vi "Image_Actions_V3.vi"(0 "Image Size (Pixels)":T2={"Pixels Per Line"=128, "Number of Lines"=128}, 2 "Mode":u16(ring) items=["Write", "Read"], 7 "Number of Channels":i32, 11 "Action":string) -> (4 "Image REFs OUT":T1[](array[typedef]), 15 "Image Names OUT":string[](array[string]))   [LabVIEW 2014]
uses:
  <vilib>/vision/Image Controls.llb/IMAQ Image.ctl
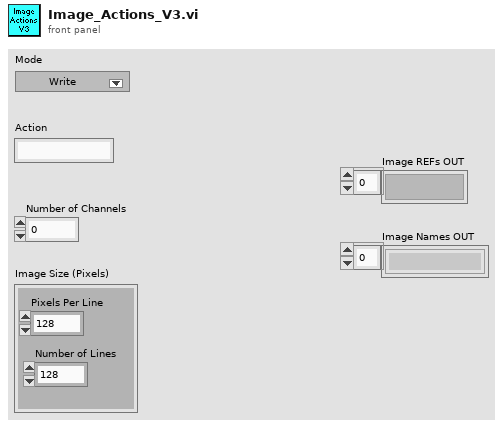
[diagram p1: front panel]
types:
  T1 = typedef "IMAQ Image.ctl" = refnum<image>
  T2 = cluster{"Pixels Per Line":i32, "Number of Lines":i32}
  T3 = typedef "Image Type" = u32
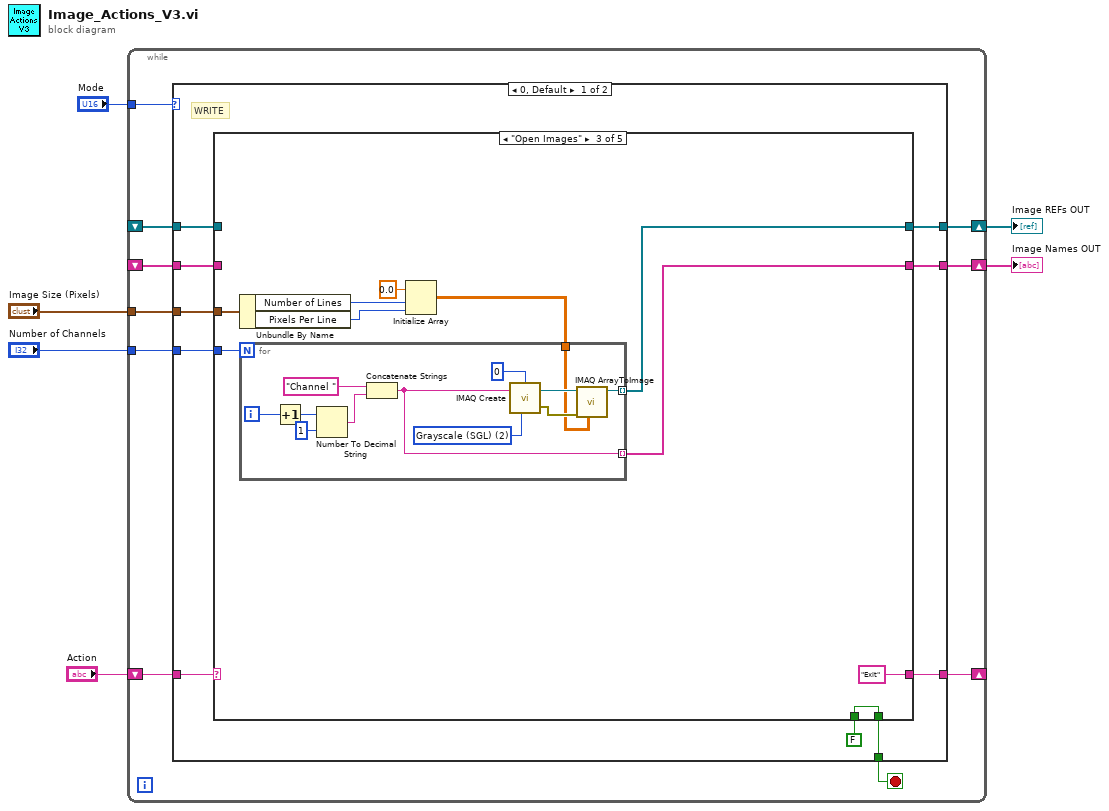
[diagram p0: block diagram]
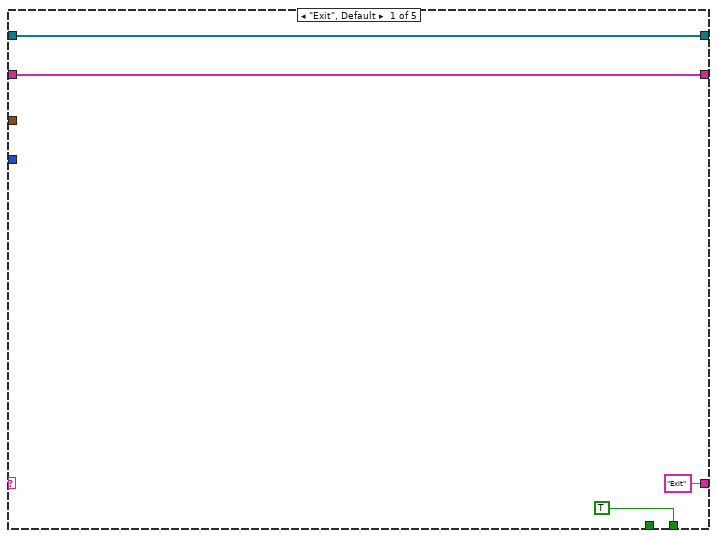
[diagram p2: hidden frame]
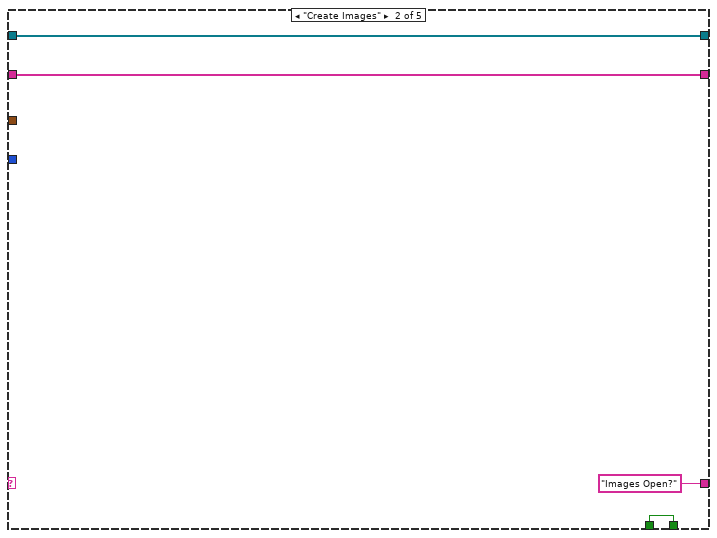
[diagram p3: hidden frame]
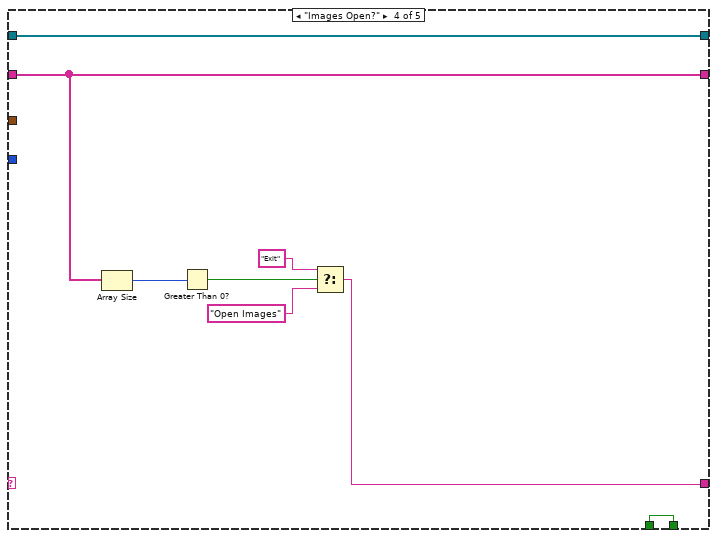
[diagram p4: hidden frame]
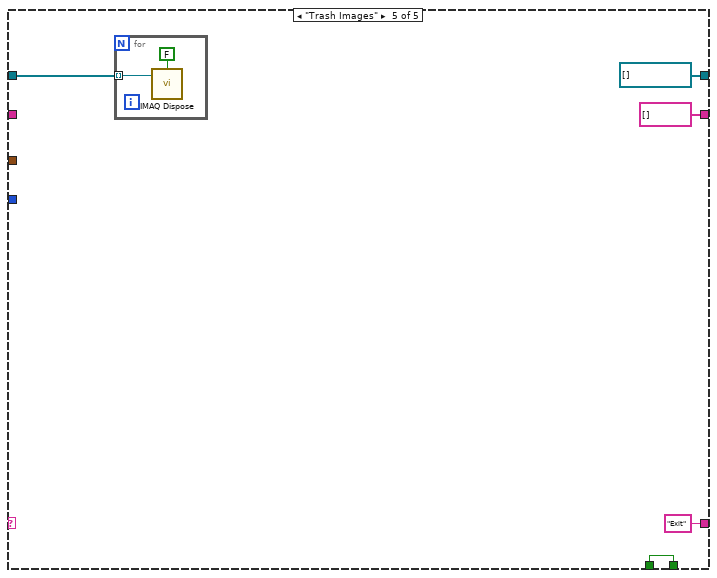
[diagram p5: hidden frame]
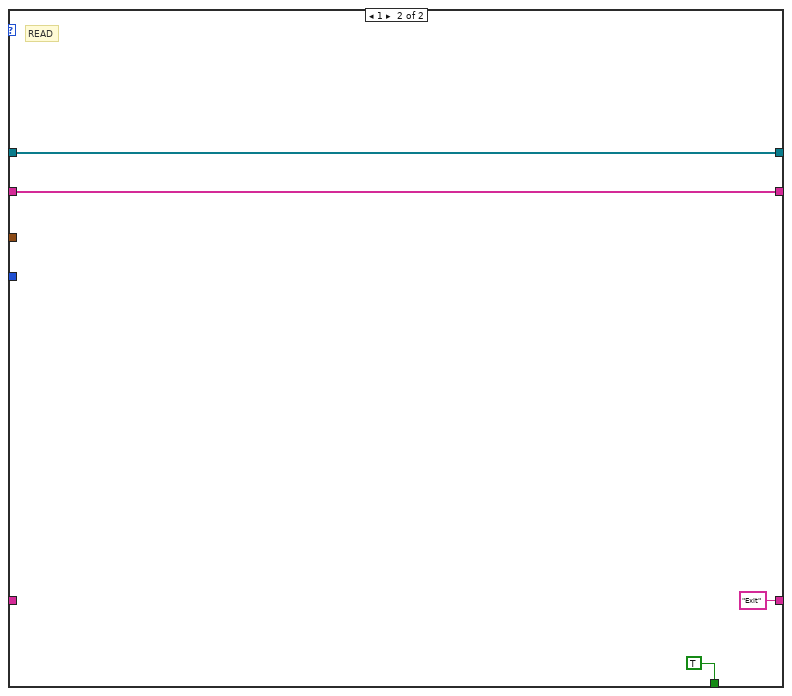
[diagram p6: hidden frame]
diagram:
  n1 = while {
    tunnel: "Mode" -> [w16]
    shift-right: [w7] -> _
    shift-left: "Action" -> [w14]
    shift-right: [w11] -> w2
    shift-left: _ -> [w9]
    tunnel: "Number of Channels" -> [w13]
    tunnel: "Image Size (Pixels)" -> [w12]
    shift-right: [w10] -> w1
    shift-left: _ -> [w8]
    stop <- w15 stop-if-true
    n2 = case shown="0, Default" w16 {
      tunnel: [w21 TRUE] -> w15
      tunnel: w14 -> [w26 _]
      tunnel: w13 -> [w25 _]
      tunnel: w12 -> [w24 _]
      tunnel: [w23 w74] -> w11
      tunnel: [w22 w73] -> w10
      tunnel: w9 -> [w18 w74]
      tunnel: w8 -> [w17 w73]
      tunnel: [w19 "Exit"] -> w7
      frame 0, Default {
        # "WRITE"
        n3 = case shown="\"Open Images\"" w26 {
          tunnel: w25 -> [_ _ w44 _ _]
          tunnel: w24 -> [_ _ w43 _ _]
          tunnel: [w28 w32 w38 w63 T1[] []] -> w23
          tunnel: [w27 w31 w37 w62 string[] []] -> w22
          tunnel: [TRUE w34 w36 w64 w67] -> w21
          tunnel: FALSE -> [_ w34 w36 w64 w67]
          tunnel: ["Exit" "Images Open?" "Exit" w59 "Exit"] -> w19
          tunnel: w18 -> [w28 w32 _ w63 w65]
          tunnel: w17 -> [w27 w31 _ w62 _]
          frame "Exit", Default {
          }
          frame "Create Images" {
          }
          frame "Open Images" {
            n4 = Unbundle By Name(w43) -> ("Number of Lines"=w41:i32, "Pixels Per Line"=w42:i32)
            n5 = Initialize Array(sgl 0.0 ("element"), w41, w42) -> (w39:sgl[][])
            n6 = for {
              N: w44 -> [_]
              tunnel: w39 -> [w48]
              tunnel: [w46] -> w38 mode=indexing
              tunnel: [w45] -> w37 mode=indexing
              i -> [w47]
              w52 = T3 2 items=["Grayscale (U8)", "Grayscale (I16)", "Grayscale (SGL)", "Complex (CSG)", "RGB (U32)", "HSL (U32)", "RGB (U64)", "Grayscale (U16)"] ("Image Type")
              n7 = Increment(x=w47) -> (x+1=w54:i32)
              n8 = Number To Decimal String(number=w54, width (-)=i16 1) -> (decimal integer string=w51:string)
              n9 = Concatenate Strings("Channel ", w51) -> (w45:string)
              n10 = call "IMAQ Create"("Border Size"=0, "Image Name"=w45, "Image Type"=w52) -> ("New Image"=w53:T1, "error out"=w56:errorcluster)  [unwired: 2 in]
              n11 = call "IMAQ ArrayToImage"("Image Pixels (Float)"=w48, "error in (no error)"=w56, "Image"=w53) -> ("Image Out"=w46:T1)  [unwired: 7 in, 1 out]
            }
          }
          frame "Images Open?" {
            n12 = Array Size(array=w62) -> (size(s)=w61:i32)
            n13 = Greater Than 0?(x=w61) -> (x > 0?=w60:bool)
            n14 = Select(t="Exit", s=w60, f="Open Images") -> (s? t:f=w59:string)
          }
          frame "Trash Images" {
            n15 = for {
              tunnel: w65 -> [w71] mode=indexing
              n16 = call "IMAQ Dispose"("All Images? (No)"=FALSE, "Image"=w71) -> ()  [unwired: 4 in, 1 out]
            }
          }
        }
      }
      frame 1 {
        # "READ"
      }
    }
  }
  "Image REFs OUT" <- w2
  "Image Names OUT" <- w1
